vi "GitPull.vi"(8 "error in (no error)":errorcluster, 11 "Directory (leave empty for relative)":path) -> (0 "error out":errorcluster, 3 "directory out":path=path "C:/RageATE/Labview Utilities/GitTools", 5 "Git Ok?(t)":bool)   [LabVIEW 2018]
panel:
  out "Numeric":i32
  out "standard error":string="POST git-upload-pack (154 bytes)\nFrom https://github.com/RaGESystemsCGH/RageATE\n   e4d4f6d6..d921aa86  main       -> origin/main\n"
  out "standard output":string="!!!SW is not up to date with origin on server.\nCheck the message and correct the issue using Github!!\n\n\nPOST git-upload-pack (154 bytes)\nFrom https://github.com/RaGESystemsCGH/RageATE\n   e4d4f6d6..d921aa86  main       -> origin/main\n"
  out "git status":string[](array[string])=["POST git-upload-pack (154 bytes)", "From https://github.com/RaGESystemsCGH/RageATE", "   e4d4f6d6..d921aa86  main       -> origin/main"]
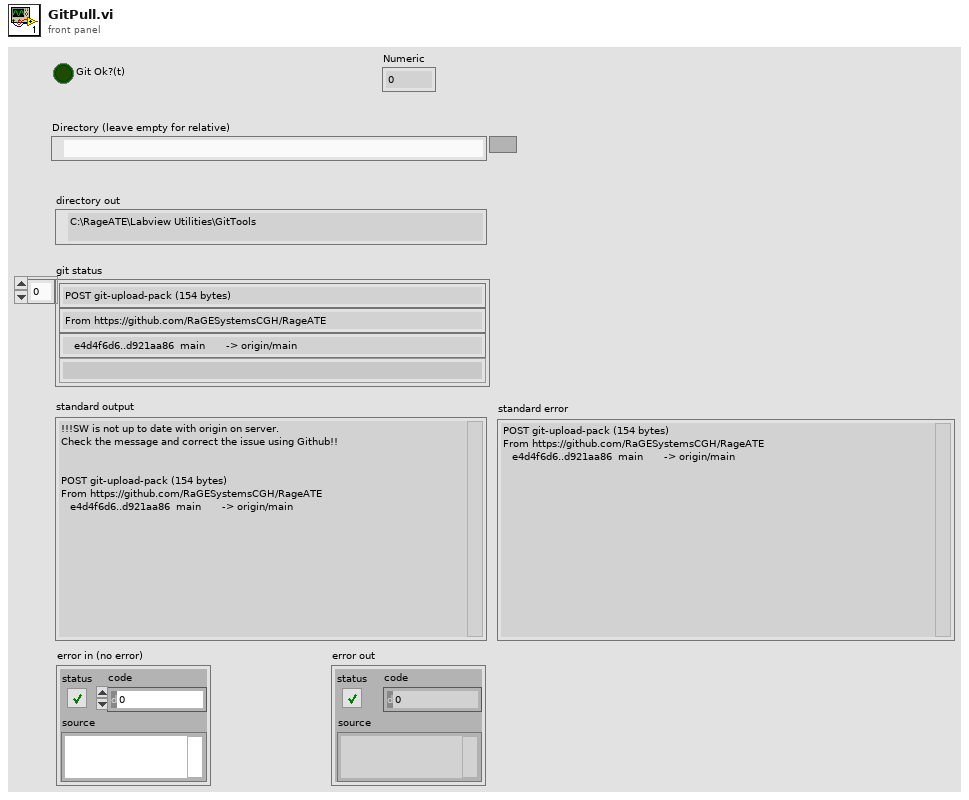
[diagram p1: front panel]
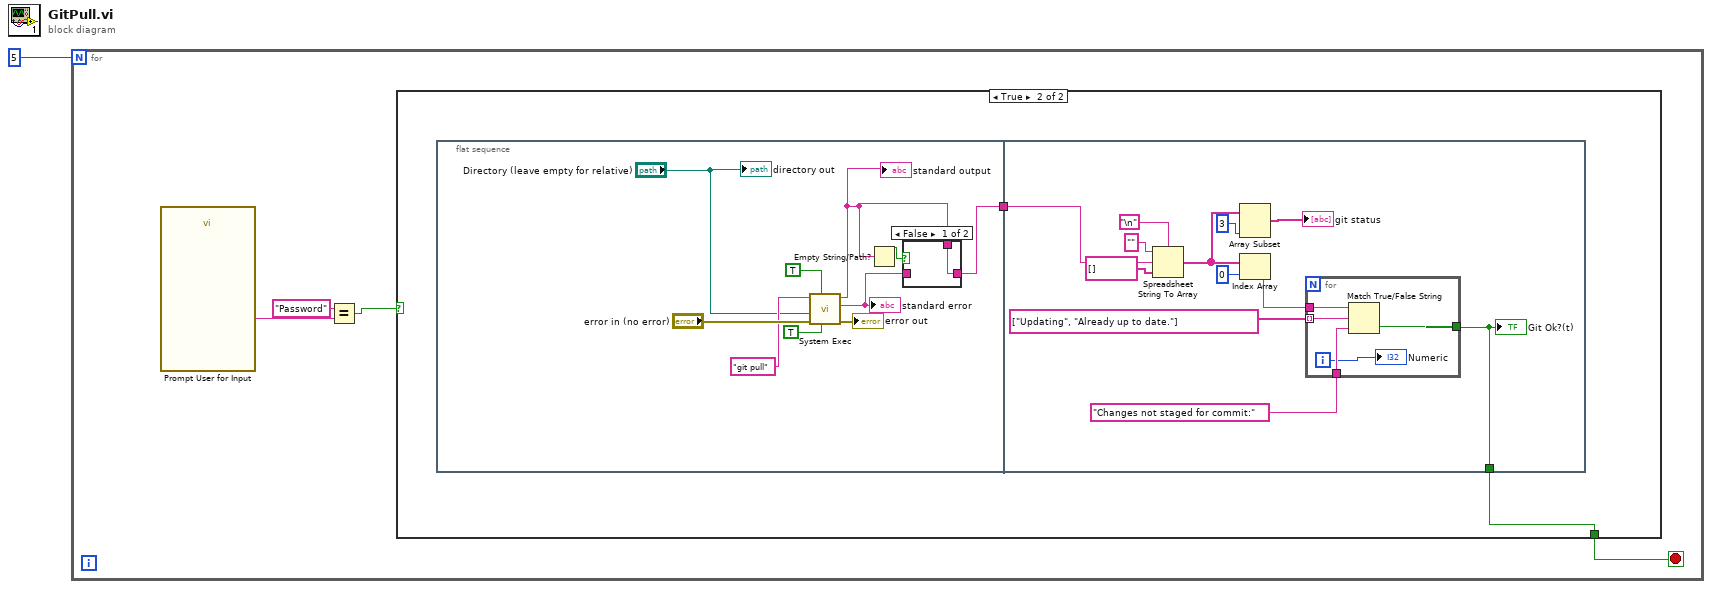
[diagram p0: block diagram]
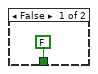
[diagram p2: hidden frame]
diagram:
  n1 = for {
    N: 5 -> [_]
    stop <- w2 stop-if-true
    n2 = call "Prompt User for Input"() -> ("Enter PW"=w5:string)  [unwired: 17 in, 2 out]
    n3 = Equal?(x="Password", y=w5) -> (x = y?=w3:bool)
    n4 = case shown="True" w3 {
      tunnel: [FALSE ("stop") w7] -> w2
      frame False {
      }
      frame True {
        n5 = flat-sequence {
          tunnel: [w12] -> w8
          tunnel: w8 -> [w22]
          tunnel: [w21] -> w7
          frame #0 {
            n6 = call <vilib>:"System Exec.vi"("run minimized? (F)"=TRUE, "wait until completion? (T)"=TRUE, "error in (no error)"="error in (no error)", "working directory"="Directory (leave empty for relative)", "command line"="git pull") -> ("error out"=→"error out":errorcluster, "standard error"=w11:string, "standard output"=w9:string)  [unwired: 3 in, 1 out]
            "standard error" <- w11
            "standard output" <- w9
            n7 = Empty String/Path?(string/path=w9) -> (empty?=w13:bool)
            n8 = case shown="False" w13 {
              tunnel: [w19 w20] -> w12
              tunnel: w11 -> [_ w20]
              tunnel: w9 -> [w19 _]
              frame False {
              }
              frame True {
              }
            }
            "directory out" <- "Directory (leave empty for relative)"
          }
          frame #1 {
            n9 = Spreadsheet String To Array(delimiter (Tab)="\n", format string="", spreadsheet string=w22, array type (2D Dbl)=string[] []) -> (array=w31:string[])
            n10 = Array Subset(array=w31, length=3) -> (→"git status":string[])  [unwired: 1 in]
            n11 = Index Array(array=w31, index=0) -> (element=w32:string)
            n12 = for {
              tunnel: [w37] -> w21
              tunnel: w32 -> [w36]
              tunnel: "Changes not staged for commit:" ("false string") -> [w35]
              tunnel: string[] ["Updating", "Already up to date."] ("false string") -> [w34] mode=indexing
              i -> [w33]
              n13 = Match True/False String(2:w35, 3:w34, 4:w36) -> (0:w37:bool)  [unwired: 1 out]
              "Numeric" <- w33
            }
            "Git Ok?(t)" <- w21
          }
        }
      }
    }
  }
